vi "connection_example.vi"(0 "Numeric 3":dbl, 1 "Numeric 2":dbl, 3 "Numeric":dbl) -> (2 "Numeric 4":dbl)   [LabVIEW 2017]
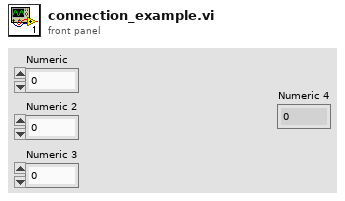
[diagram p1: front panel]
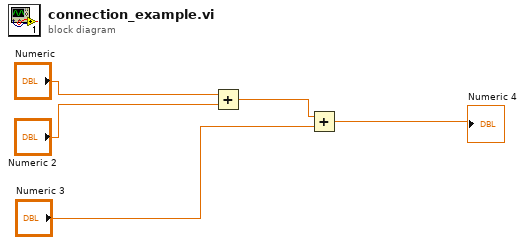
[diagram p0: block diagram]
diagram:
  n1 = Add(x="Numeric", y="Numeric 2") -> (x+y=w3:dbl)
  n2 = Add(x=w3, y="Numeric 3") -> (x+y=→"Numeric 4":dbl)
